vi "DesignPatterns_GeneratePatternFile.vi"(0 "FilePath":path, 1 "Pattern":T1, 2 "Nodes":T2[](array[typedef]), 3 "Links":T4[](array[typedef]), 5 "error in (no error)":errorcluster, 6 "UseWikiHelpUrl(True)":bool=TRUE) -> (15 "StringOut":string, 19 "error out":errorcluster)   [LabVIEW 2010]
uses:
  DesignPatterns_Link.ctl
  DesignPatterns_LinkType.ctl
  DesignPatterns_Node.ctl
  DesignPatterns_NodeType.ctl
  DesignPatterns_Pattern.ctl
  DesignPatterns_ClassNodeData.ctl
  DesignPatterns_Attribute.ctl
  DesignPatterns_Method.ctl
  DesignPatterns_NoteNodeData.ctl
  DesignPatterns_NoteLink.ctl
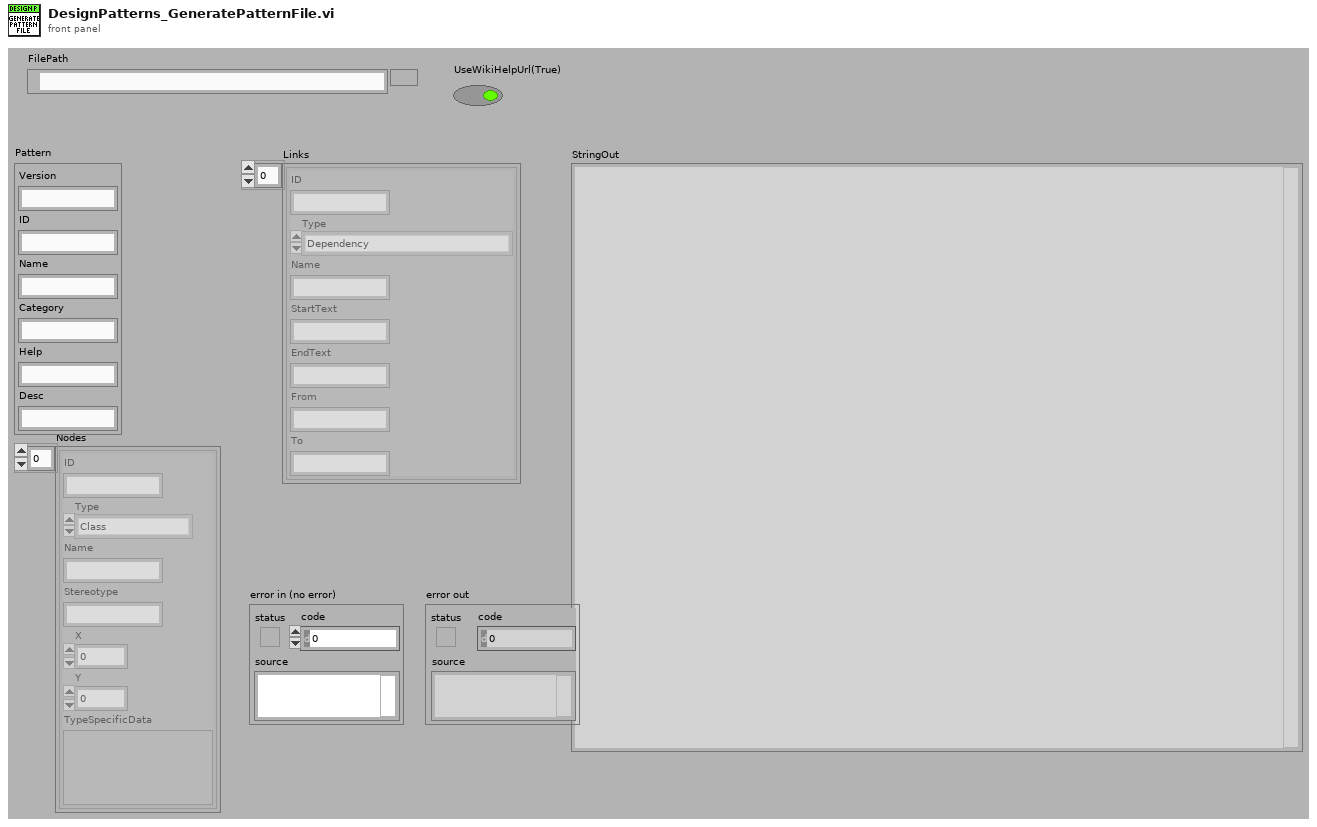
[diagram p1: front panel]
types:
  T1 = typedef "DesignPatterns_Pattern.ctl" = cluster{"Version":string, "ID":string, "Name":string, "Category":string, "Help":string, "Desc":string}
  T2 = typedef "DesignPatterns_Node.ctl" = cluster{"ID":string, "Type":T3, "Name":string, "Stereotype":string, "X":i32, "Y":i32, "TypeSpecificData":variant}
  T3 = typedef "DesignPatterns_NodeType.ctl" = enum16{"Class", "Interface", "Note", "Package"}
  T4 = typedef "DesignPatterns_Link.ctl" = cluster{"ID":string, "Type":T5, "Name":string, "StartText":string, "EndText":string, "From":string, "To":string}
  T5 = typedef "DesignPatterns_LinkType.ctl" = enum16{"Dependency", "Inheritance", "Interface", "Association", "Aggregation", "CompositeAggregation"}
  T6 = typedef "DesignPatterns_ClassNodeData.ctl" = cluster{"Description":string, "Attributes":T7[], "Methods":T8[]}
  T7 = typedef "DesignPatterns_Attribute.ctl" = cluster{"ID":string, "Name":string}
  T8 = typedef "DesignPatterns_Method.ctl" = cluster{"ID":string, "Name":string}
  T9 = typedef "DesignPatterns_NoteNodeData.ctl" = cluster{"Text":string, "Links":T10[]}
  T10 = typedef "DesignPatterns_NoteLink.ctl" = cluster{"ID":string, "source":string}
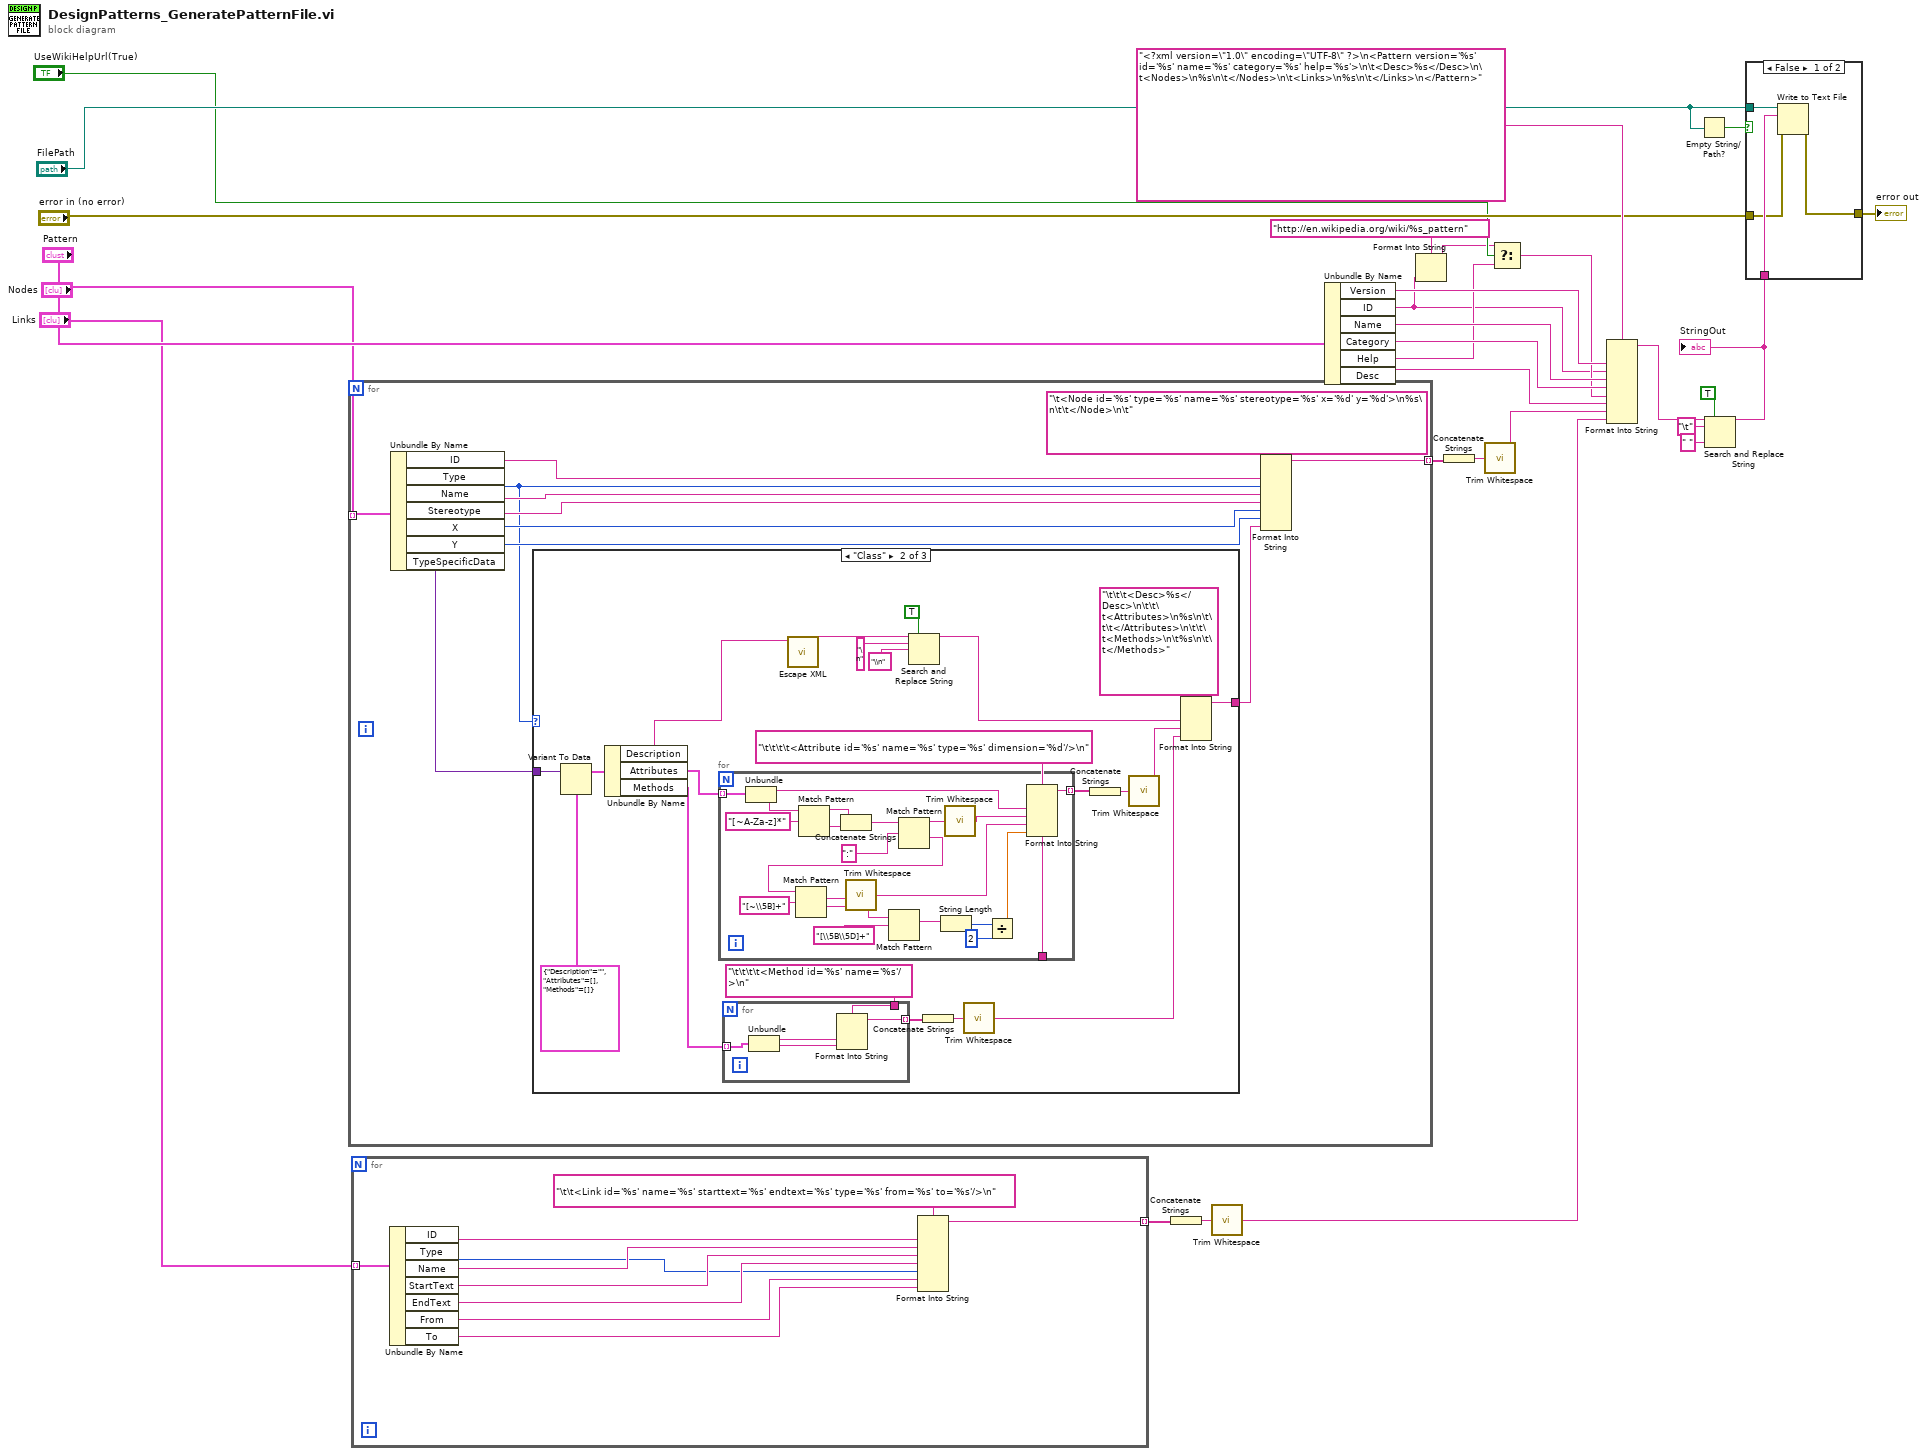
[diagram p0: block diagram]
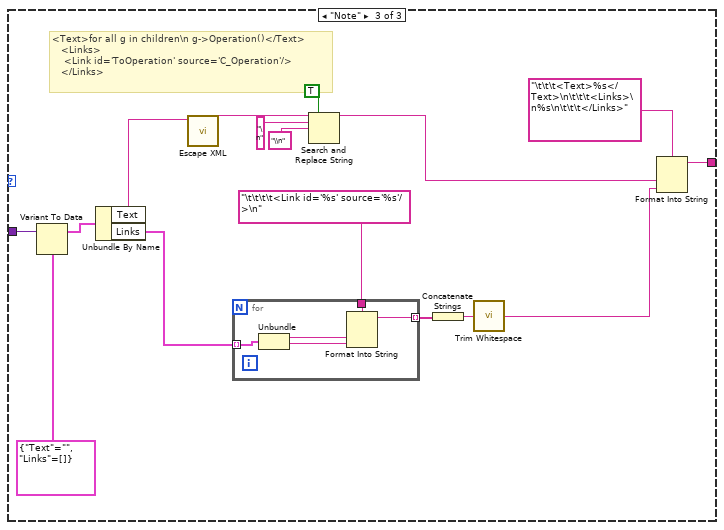
[diagram p4: hidden frame]
diagram:
  n1 = for {
    tunnel: "Nodes" -> [w40] mode=indexing
    tunnel: [w30] -> w25 mode=indexing
    n2 = Unbundle By Name(w40) -> ("ID"=w39:string, "Type"=w33:T3, "Name"=w38:string, "Stereotype"=w37:string, "X"=w36:i32, "Y"=w35:i32, "TypeSpecificData"=w34:variant)
    n3 = case shown="\"Class\"" w33 {
      tunnel: w34 -> [_ w61 w104]
      tunnel: [_ w47 w98] -> w32
      frame Default {
      }
      frame "Class" {
        n4 = Variant To Data(Variant=w61, type=T6 {"Description"="", "Attributes"=[], "Methods"=[]} ("ClassSpecificData")) -> (data=w59:T6)  [unwired: 1 in, 1 out]
        n5 = Unbundle By Name(w59) -> ("Description"=w42:string, "Attributes"=w57:T7[], "Methods"=w52:T8[])
        n6 = for {
          tunnel: w57 -> [w88] mode=indexing
          tunnel: "\t\t\t\t<Attribute id='%s' name='%s' type='%s' dimension='%d'/>\n" ("Description") -> [w87]
          tunnel: [w68] -> w55 mode=indexing
          n7 = Unbundle(w88) -> ("ID"=w86:string, "Name"=w85:string)
          n8 = Match Pattern(string=w85, regular expression="[~A-Za-z]*") -> (before substring=w67:string, after substring=w83:string)  [unwired: 3 out]
          n9 = Concatenate Strings(w67, w83) -> (w82:string)
          n10 = Match Pattern(string=w82, regular expression=":") -> (before substring=w80:string, after substring=w78:string)  [unwired: 3 out]
          n11 = Match Pattern(string=w78, regular expression="[~\\5B]+") -> (match substring=w76:string, after substring=w74:string)  [unwired: 3 out]
          n12 = call <vilib>:"Trim Whitespace.vi"("string"=w76) -> ("trimmed string"=w75:string)  [unwired: 1 in]
          n13 = Match Pattern(string=w74, regular expression="[\\5B\\5D]+") -> (match substring=w72:string)  [unwired: 4 out]
          n14 = String Length(string=w72) -> (length=w71:i32)
          n15 = call <vilib>:"Trim Whitespace.vi"("string"=w80) -> ("trimmed string"=w79:string)  [unwired: 1 in]
          n16 = Divide(x=w71, y=2) -> (x/y=w69:dbl)
          n17 = Format Into String(format string=w87, w86, w79, w75, w69) -> (resulting string=w68:string)  [unwired: 2 in, 1 out]
        }
        n18 = for {
          tunnel: w52 -> [w66] mode=indexing
          tunnel: "\t\t\t\t<Method id='%s' name='%s'/>\n" ("Description") -> [w65]
          tunnel: [w62] -> w49 mode=indexing
          n19 = Unbundle(w66) -> ("ID"=w64:string, "Name"=w63:string)
          n20 = Format Into String(format string=w65, w64, w63) -> (resulting string=w62:string)  [unwired: 2 in, 1 out]
        }
        n21 = call <vilib>:"Escape XML.vi"("XML String In"=w42) -> ("XML String Out"=w44:string)  [unwired: 1 in, 9 out]
        n22 = Search and Replace String(replace all?=TRUE ("replace all? (F)"), input string=w44, search string="\n" ("replace string (\"\")"), replace string="\\n" ("search string")) -> (result string=w41:string)  [unwired: 1 in, 6 out]
        n23 = Concatenate Strings(w49) -> (w50:string)
        n24 = call <vilib>:"Trim Whitespace.vi"("string"=w50) -> ("trimmed string"=w48:string)  [unwired: 1 in]
        n25 = Concatenate Strings(w55) -> (w54:string)
        n26 = call <vilib>:"Trim Whitespace.vi"("string"=w54) -> ("trimmed string"=w53:string)  [unwired: 1 in]
        n27 = Format Into String(format string="\t\t\t<Desc>%s</Desc>\n\t\t\t<Attributes>\n%s\n\t\t\t</Attributes>\n\t\t\t<Methods>\n\t%s\n\t\t</Methods>" ("Description"), w41, w53, w48) -> (resulting string=w47:string)  [unwired: 2 in, 1 out]
      }
      frame "Note" {
        # "<Text>for all g in children\\n g->Operation()</Text>\n\t\t\t<Links>\n\t\t\t\t<Link id='ToOperation' source='C_Operation'/>\n\t\t\t</Links>"
        n28 = Variant To Data(Variant=w104, type=T9 {"Text"="", "Links"=[]} ("NoteNodeData")) -> (data=w102:T9)  [unwired: 1 in, 1 out]
        n29 = Unbundle By Name(w102) -> ("Text"=w93:string, "Links"=w91:T10[])
        n30 = call <vilib>:"Escape XML.vi"("XML String In"=w93) -> ("XML String Out"=w96:string)  [unwired: 1 in, 9 out]
        n31 = for {
          tunnel: w91 -> [w109] mode=indexing
          tunnel: "\t\t\t\t<Link id='%s' source='%s'/>\n" ("Description") -> [w108]
          tunnel: [w105] -> w99 mode=indexing
          n32 = Unbundle(w109) -> ("ID"=w107:string, "source"=w106:string)
          n33 = Format Into String(format string=w108, w107, w106) -> (resulting string=w105:string)  [unwired: 2 in, 1 out]
        }
        n34 = Search and Replace String(replace all?=TRUE ("replace all? (F)"), input string=w96, search string="\n" ("replace string (\"\")"), replace string="\\n" ("search string")) -> (result string=w92:string)  [unwired: 1 in, 6 out]
        n35 = Concatenate Strings(w99) -> (w100:string)
        n36 = call <vilib>:"Trim Whitespace.vi"("string"=w100) -> ("trimmed string"=w89:string)  [unwired: 1 in]
        n37 = Format Into String(format string="\t\t\t<Text>%s</Text>\n\t\t\t<Links>\n%s\n\t\t\t</Links>" ("Description"), w92, w89) -> (resulting string=w98:string)  [unwired: 2 in, 1 out]
      }
    }
    n38 = Format Into String(format string="\t<Node id='%s' type='%s' name='%s' stereotype='%s' x='%d' y='%d'>\n%s\n\t\t</Node>\n\t", w39, w33, w38, w37, w36, w35, w32) -> (resulting string=w30:string)  [unwired: 2 in, 1 out]
  }
  n39 = for {
    tunnel: "Links" -> [w119] mode=indexing
    tunnel: [w110] -> w28 mode=indexing
    n40 = Unbundle By Name(w119) -> ("ID"=w117:string, "Type"=w113:T5, "Name"=w116:string, "StartText"=w115:string, "EndText"=w114:string, "From"=w112:string, "To"=w111:string)
    n41 = Format Into String(format string="\t\t<Link id='%s' name='%s' starttext='%s' endtext='%s' type='%s' from='%s' to='%s'/>\n", w117, w116, w115, w114, w113, w112, w111) -> (resulting string=w110:string)  [unwired: 2 in, 1 out]
  }
  n42 = Concatenate Strings(w28) -> (w27:string)
  n43 = call <vilib>:"Trim Whitespace.vi"("string"=w27) -> ("trimmed string"=w29:string)  [unwired: 1 in]
  n44 = Unbundle By Name("Pattern") -> ("Version"=w19:string, "ID"=w8:string, "Name"=w20:string, "Category"=w21:string, "Help"=w10:string, "Desc"=w22:string)
  n45 = Format Into String(format string="http://en.wikipedia.org/wiki/%s_pattern", w8) -> (resulting string=w6:string)  [unwired: 2 in, 1 out]
  n46 = Concatenate Strings(w25) -> (w24:string)
  n47 = call <vilib>:"Trim Whitespace.vi"("string"=w24) -> ("trimmed string"=w26:string)  [unwired: 1 in]
  n48 = Select(t=w6, s="UseWikiHelpUrl(True)", f=w10) -> (s? t:f=w11:string)
  n49 = Format Into String(format string="<?xml version=\"1.0\" encoding=\"UTF-8\" ?>\n<Pattern version='%s' id='%s' name='%s' category='%s' help='%s'>\n\t<Desc>%s</Desc>\n\t<Nodes>\n%s\n\t</Nodes>\n\t<Links>\n%s\n\t</Links>\n</Pattern>", w19, w8, w20, w21, w11, w22, w26, w29) -> (resulting string=w2:string)  [unwired: 2 in, 1 out]
  n50 = Empty String/Path?(string/path="FilePath") -> (empty?=w13:bool)
  n51 = Search and Replace String(replace all?=TRUE ("replace all? (F)"), input string=w2, search string="\t", replace string=" " ("replace string (\"\")")) -> (result string=w1:string)  [unwired: 1 in, 6 out]
  "StringOut" <- w1
  n52 = case shown="False" w13 {
    tunnel: [w123 w124] -> w15
    tunnel: "FilePath" -> [w122 _]
    tunnel: w1 -> [w121 _]
    tunnel: "error in (no error)" -> [w120 w124]
    frame False {
      n53 = Write to Text File(file (use dialog)=w122, text=w121, error in=w120) -> (error out=w123:errorcluster)  [unwired: 3 out]
    }
    frame True {
    }
  }
  "error out" <- w15
